vi "Test Add to Child List.vi"(8 "error in (no error)":errorcluster) -> (0 "error out":errorcluster)   [LabVIEW 2017, in "Unit Tests.lvlib"]
uses:
  Unit Tests.lvlib
  source/Browser Core/Node Classes/Generic Node/Generic Node.lvclass
  source/Browser Core/Node Classes/Generic Node/Generic Node.lvclass/Generic Node.ctl
  <vilib>/addons/_JKI Toolkits/Caraya/classes/Test/Test.lvclass
  <vilib>/addons/_JKI Toolkits/Caraya/classes/Assert/Assert.lvclass
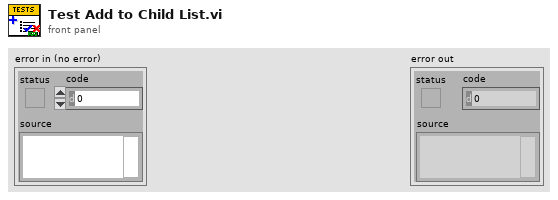
[diagram p1: front panel]
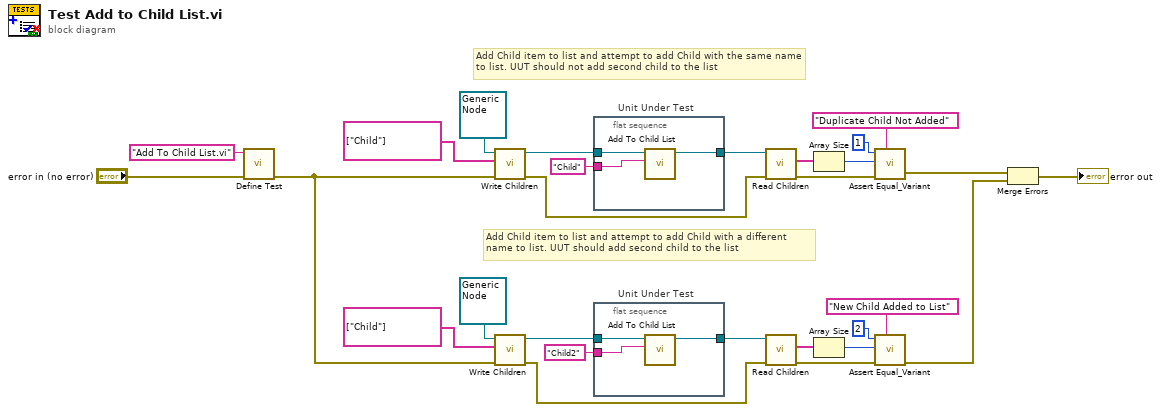
[diagram p0: block diagram]
diagram:
  # "Add Child item to list and attempt to add Child with a different name to list. UUT should add second child to the list"
  # "Add Child item to list and attempt to add Child with the same name to list. UUT should not add second child to the list"
  n1 = call <vilib>:"Define Test.vi"("error in (no error)"="error in (no error)", "Label (VI Title)"="Add To Child List.vi") -> ("error out"=w4:errorcluster)  [unwired: 9 in]
  n2 = call "Write Children.vi"("error in (no error)"=w4, "Children"=string[] ["Child"], "Generic Node in"=refnum<class "Generic Node.lvclass"> refnum ("Browser Core.lvlib:Generic Node.lvclass")) -> ("error out"=w22:errorcluster, "Generic Node out"=w28:refnum<class "Generic Node.lvclass">)  [unwired: 7 in]
  n3 = call "Write Children.vi"("error in (no error)"=w4, "Children"=string[] ["Child"], "Generic Node in"=refnum<class "Generic Node.lvclass"> refnum ("Browser Core.lvlib:Generic Node.lvclass")) -> ("error out"=w10:errorcluster, "Generic Node out"=w5:refnum<class "Generic Node.lvclass">)  [unwired: 7 in]
  n4 = flat-sequence "Unit Under Test" {
    tunnel: w28 -> [w31]
    tunnel: [w30] -> w26
    tunnel: "Child" ("UID") -> [w29]
    frame #0 {
      n5 = call-dynamic "Add To Child List.vi"("Child ID"=w29, "Generic Node in"=w31) -> ("Generic Node out"=w30:refnum<class "Generic Node.lvclass">)  [unwired: 9 in]
    }
  }
  n6 = flat-sequence "Unit Under Test" {
    tunnel: w5 -> [w34]
    tunnel: [w33] -> w7
    tunnel: "Child2" ("UID") -> [w32]
    frame #0 {
      n7 = call-dynamic "Add To Child List.vi"("Child ID"=w32, "Generic Node in"=w34) -> ("Generic Node out"=w33:refnum<class "Generic Node.lvclass">)  [unwired: 9 in]
    }
  }
  n8 = call "Read Children.vi"("error in (no error)"=w22, "Generic Node in"=w26) -> ("error out"=w20:errorcluster, "Children"=w21:string[])  [unwired: 7 in, 1 out]
  n9 = call "Read Children.vi"("error in (no error)"=w10, "Generic Node in"=w7) -> ("error out"=w12:errorcluster, "Children"=w11:string[])  [unwired: 7 in, 1 out]
  n10 = Array Size(array=w21) -> (size(s)=w19:i32)
  n11 = Array Size(array=w11) -> (size(s)=w13:i32)
  n12 = call <vilib>:"Assert Equal_Variant.vi"("Label"="Duplicate Child Not Added", "error in (no error)"=w20, "Y"=w19, "X"=1 ("size(s)")) -> ("error out"=w3:errorcluster)  [unwired: 7 in]
  n13 = call <vilib>:"Assert Equal_Variant.vi"("Label"="New Child Added to List", "error in (no error)"=w12, "Y"=w13, "X"=2 ("size(s)")) -> ("error out"=w1:errorcluster)  [unwired: 7 in]
  n14 = Merge Errors(w3, w1) -> (→"error out":errorcluster)
